vi "Step DAO.vi"(8 "error in (no error)":errorcluster, 9 "Step Count In":string, 10 "Step In":T1[](array[typedef]), 11 "Step DAO Actions":T3) -> (0 "error out":errorcluster, 1 "Step Count Out":string, 2 "Step Out":T1[](array[typedef]), 3 "Start Time":timestamp, 5 "Duplicates found":bool)   [LabVIEW 2009]
uses:
  Target.ctl
  Data Access Objects/Metadata/LBCB Number.ctl
  Step DAO Actions.ctl
panel:
  in  "Default Initial Step":T1[](array[typedef])=[{"LBCB Number"=enum."LBCB1", "DOF Vectors"=enum."Dx", "Amount"=0.0}, {"LBCB Number"=enum."LBCB1", "DOF Vectors"=enum."Dy", "Amount"=0.0}, {"LBCB Number"=enum."LBCB1", "DOF Vectors"=enum."Dz", "Amount"=0.0}, {"LBCB Number"=enum."LBCB2", "DOF Vectors"=enum."Dx", "Amount"=0.0}, {"LBCB Number"=enum."LBCB2", "DOF Vectors"=enum."Dy", "Amount"=0.0}, {"LBCB Number"=enum."LBCB2", "DOF Vectors"=enum."Dz", "Amount"=0.0}]
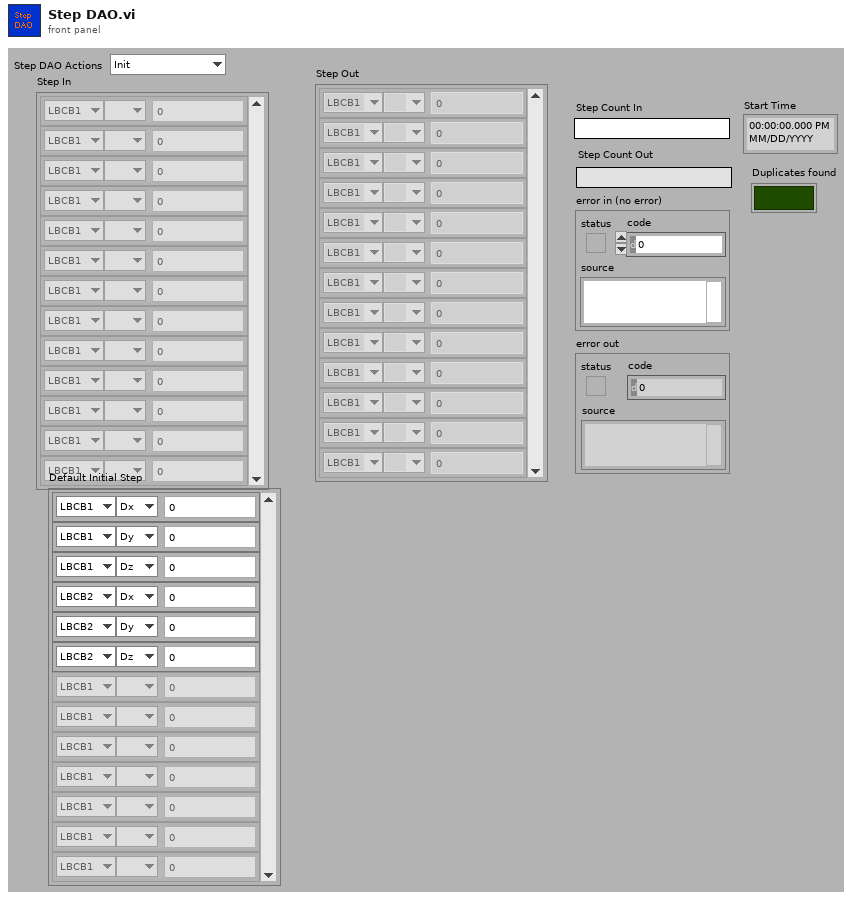
[diagram p1: front panel]
types:
  T1 = typedef "Target.ctl" = cluster{"LBCB Number":T2, "DOF Vectors":enum16{" ", "Dx", "Dy", "Dz", "Rx", "Ry", "Rz", "Fx", "Fy", "Fz", "Mx", "My", "Mz"}, "Amount":dbl}
  T2 = typedef "LBCB Number.ctl" = enum16{"LBCB1", "LBCB2"}
  T3 = typedef "Step DAO Actions.ctl" = enum16{"Init", "Set", "Get", "Reset Count"}
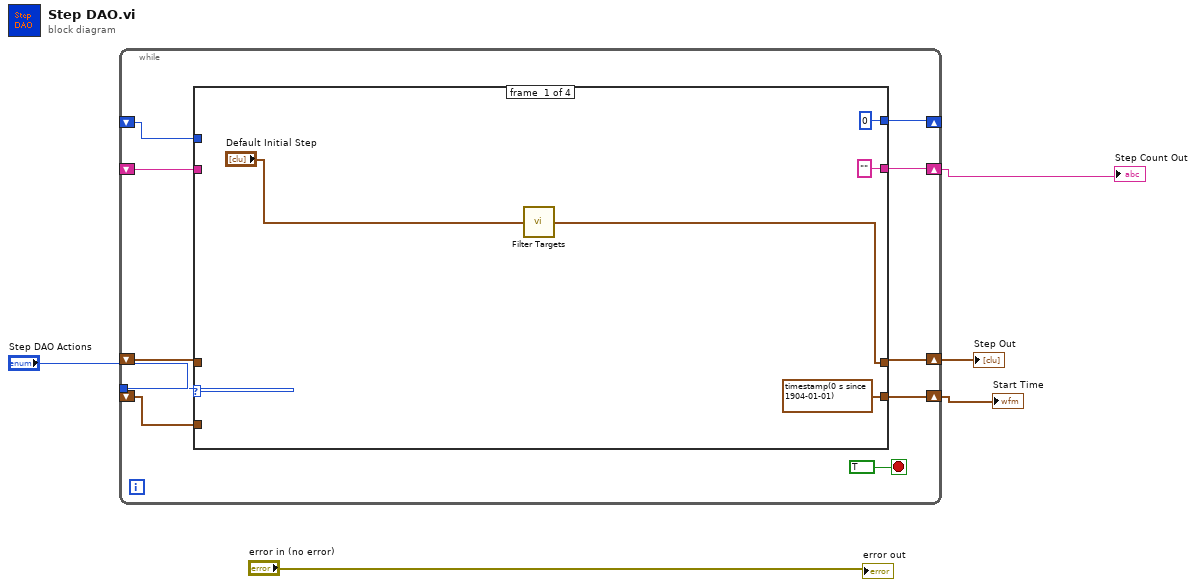
[diagram p0: block diagram]
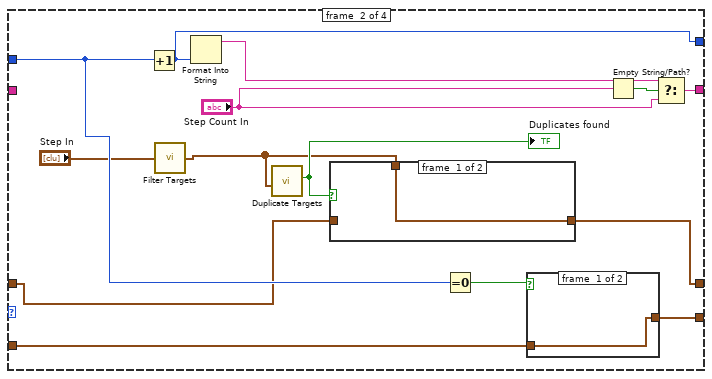
[diagram p2: hidden frame]
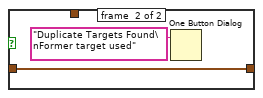
[diagram p3: hidden frame]
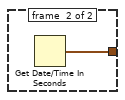
[diagram p4: hidden frame]
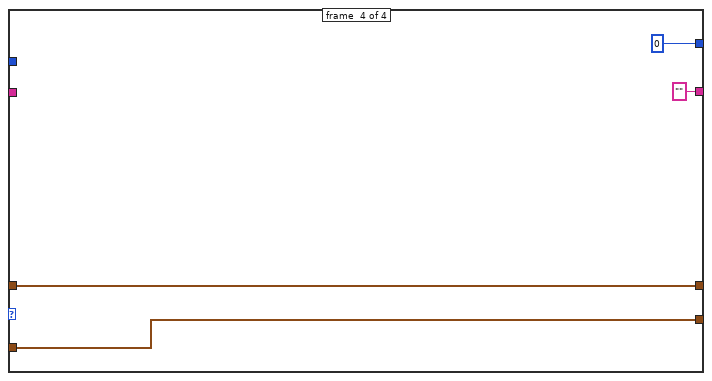
[diagram p6: hidden frame]
diagram:
  n1 = while {
    tunnel: "Step DAO Actions" -> [w14]
    shift-right: [w13] -> w4
    shift-left: _ -> [w12]
    shift-right: [w10] -> w2
    shift-left: _ -> [w8]
    shift-right: [w11] -> _
    shift-left: _ -> [w9]
    shift-right: [w7] -> w1
    shift-left: _ -> [w6]
    stop <- TRUE stop-if-true
    n2 = case shown="\"Set\"" w14 {
      tunnel: [w16 w23 w43 w45] -> w13
      tunnel: w12 -> [_ w24 w43 w45]
      tunnel: [0 w26 w42 0] -> w11
      tunnel: ["" ("Step Count In") w32 w41 "" ("Step Count In")] -> w10
      tunnel: w9 -> [_ w30 w42 _]
      tunnel: w8 -> [_ _ w41 _]
      tunnel: [timestamp(0 s since 1904-01-01) ("seconds since 1Jan1904") w28 w40 w44] -> w7
      tunnel: w6 -> [_ w27 w40 w44]
      frame #0 {
        n3 = call "Filter Targets.vi"("Targets In"="Default Initial Step") -> ("Targets Out"=w16:T1[])
      }
      frame #1 {
        n4 = Increment(x=w30) -> (x+1=w26:i32)
        n5 = call "Filter Targets.vi"("Targets In"="Step In") -> ("Targets Out"=w21:T1[])
        n6 = Format Into String(w26) -> (resulting string=w31:string)  [unwired: 3 in, 1 out]
        n7 = call "Duplicate Targets.vi"("Array"=w21) -> ("Duplicates found"=w25:bool)  [unwired: 10 out]
        "Duplicates found" <- w25
        n8 = case shown="False" w25 {
          tunnel: w24 -> [_ w37]
          tunnel: [w35 w37] -> w23
          tunnel: w21 -> [w35 _]
          frame #0 {
          }
          frame #1 {
            n9 = One Button Dialog(message="Duplicate Targets Found\nFormer target used") -> ()  [unwired: 2 out]
          }
        }
        n10 = Equal To 0?(x=w30) -> (x = 0?=w29:bool)
        n11 = case shown="False" w29 {
          tunnel: [w38 w39] -> w28
          tunnel: w27 -> [w38 _]
          frame #0 {
          }
          frame #1 {
            n12 = Get Date/Time In Seconds() -> (seconds since 1Jan1904=w39:timestamp)
          }
        }
        n13 = Empty String/Path?(string/path="Step Count In") -> (empty?=w34:bool)
        n14 = Select(t=w31, s=w34, f="Step Count In") -> (s? t:f=w32:string)
      }
      frame #2 {
      }
      frame #3 {
      }
    }
  }
  "Step Out" <- w4
  "Step Count Out" <- w2
  "Start Time" <- w1
  "error out" <- "error in (no error)"
